vi "WSVCAP SHL FPGA LL I2C Write CLK or DATA Lines.vi"(0 "Bit In":bool, 11 "error in (no error)":errorcluster, 12 "UUT Set (0/1)":u8, 13 "Line":T1, 14 "Socket Mask":u64 format="%08x") -> (15 "error out":errorcluster)   [LabVIEW 2012]
uses:
  Type Defs/WSVCAP SHL I2C Write Line Enum.ctl
  WSVCAP SHL FPGA LL I2C Debug Global.vi
  <vilib>/eio/EIONode/EIONode.xnode
  <vilib>/rvi/eio/common/nirviEmuTemplateMethod_errors.vi
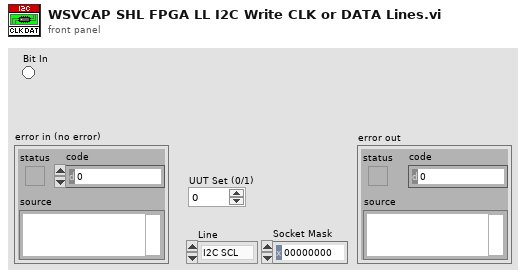
[diagram p1: front panel]
types:
  T1 = typedef "WSVCAP SHL I2C Write Line Enum.ctl" = enum16{"I2C SCL", "I2C SDA"}
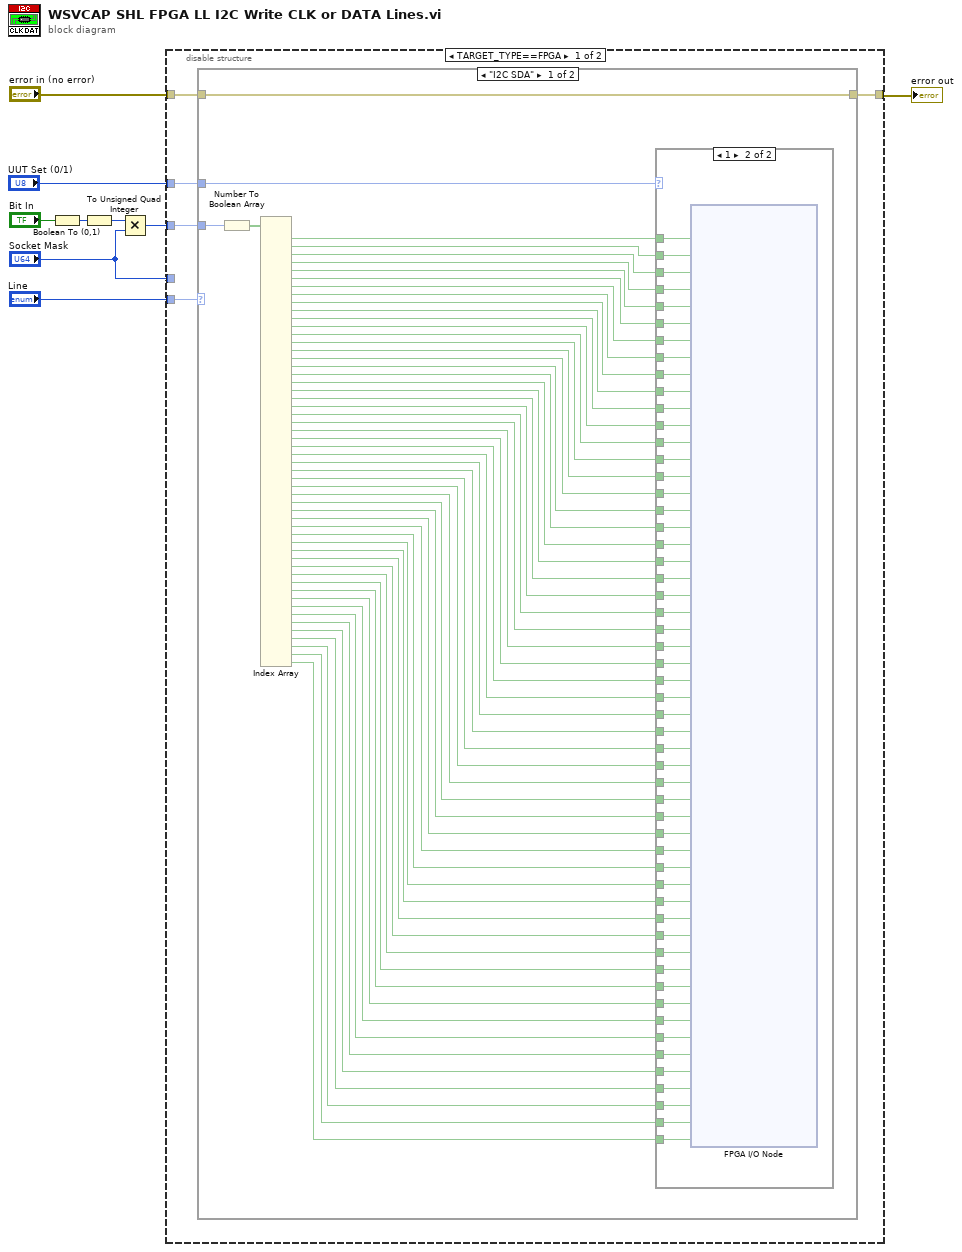
[diagram p0: block diagram]
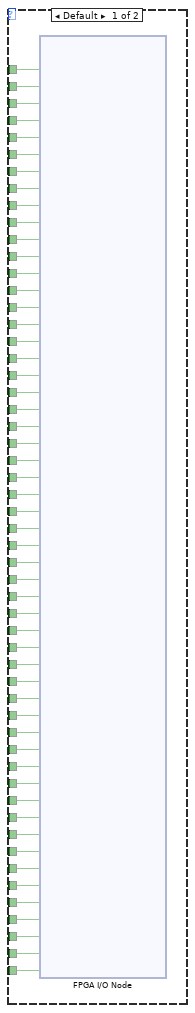
[diagram p2: hidden frame]
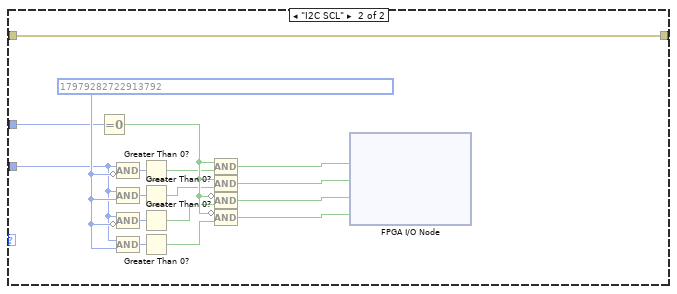
[diagram p3: hidden frame]
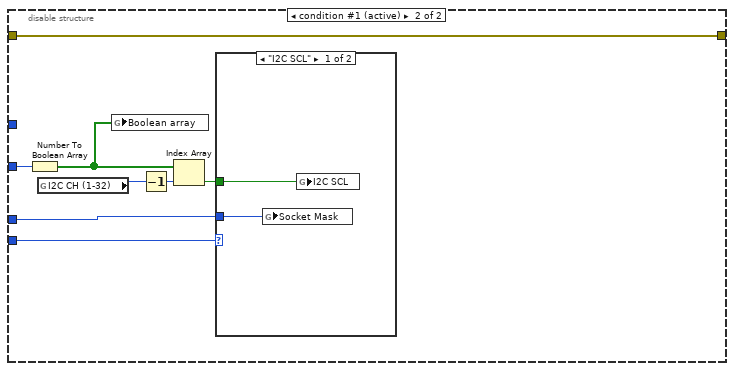
[diagram p4: hidden frame]
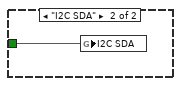
[diagram p5: hidden frame]
diagram:
  n1 = Boolean To (0,1)(Boolean="Bit In") -> (0, 1=w6:i16)
  n2 = To Unsigned Quad Integer(1:w6) -> (0:w5:u64)
  n3 = Multiply(x=w5, y="Socket Mask") -> (x*y=w3:u64)
  n4 = disable-structure shown="TARGET_TYPE==FPGA" {
    disable-tunnel: w3 -> [w14 w200]
    disable-tunnel: "Line" -> [w13 w205]
    disable-tunnel: [w12 w204] -> w8
    disable-tunnel: "error in (no error)" -> [w11 w204]
    disable-tunnel: "Socket Mask" -> [_ w198]
    disable-tunnel: "UUT Set (0/1)" -> [w10 _]
    frame condition #0 {
      n5 = case shown="\"I2C SDA\"" w13 {
        tunnel: w14 -> [w71 w185]
        tunnel: [w70 w197] -> w12
        tunnel: w11 -> [w70 w197]
        tunnel: w10 -> [w33 w186]
        frame "I2C SDA" {
          n6 = Number To Boolean Array(number=w71) -> (Boolean array=w72:bool[])
          n7 = Index Array(array=w72) -> (element #1=w69:bool, element #2=w68:bool, element #3=w67:bool, element #4=w66:bool, element #5=w65:bool, element #6=w64:bool, element #7=w63:bool, element #8=w62:bool, element #9=w61:bool, element #10=w60:bool, element #11=w59:bool, element #12=w58:bool, element #13=w57:bool, element #14=w56:bool, element #15=w55:bool, element #16=w54:bool, element #17=w53:bool, element #18=w52:bool, element #19=w51:bool, element #20=w50:bool, element #21=w49:bool, element #22=w48:bool, element #23=w47:bool, element #24=w46:bool, element #25=w45:bool, element #26=w44:bool, element #27=w43:bool, element #28=w42:bool, element #29=w41:bool, element #30=w40:bool, element #31=w39:bool, element #32=w38:bool, element #33=w37:bool, element #34=w36:bool, element #35=w35:bool, element #36=w34:bool, element #37=w32:bool, element #38=w31:bool, element #39=w30:bool, element #40=w29:bool, element #41=w28:bool, element #42=w27:bool, element #43=w26:bool, element #44=w25:bool, element #45=w24:bool, element #46=w23:bool, element #47=w22:bool, element #48=w21:bool, element #49=w20:bool, element #50=w19:bool, element #51=w18:bool, element #52=w17:bool, element #53=w16:bool, element #54=w15:bool)  [unwired: 54 in]
          n8 = case shown="1" w33 {
            tunnel: w69 -> [w126 w180]
            tunnel: w68 -> [w125 w179]
            tunnel: w67 -> [w124 w178]
            tunnel: w66 -> [w123 w177]
            tunnel: w65 -> [w122 w176]
            tunnel: w64 -> [w121 w175]
            tunnel: w63 -> [w120 w174]
            tunnel: w62 -> [w119 w173]
            tunnel: w61 -> [w118 w172]
            tunnel: w60 -> [w117 w171]
            tunnel: w59 -> [w116 w170]
            tunnel: w58 -> [w115 w169]
            tunnel: w57 -> [w114 w168]
            tunnel: w56 -> [w113 w167]
            tunnel: w55 -> [w112 w166]
            tunnel: w54 -> [w111 w165]
            tunnel: w53 -> [w110 w164]
            tunnel: w52 -> [w109 w163]
            tunnel: w51 -> [w108 w162]
            tunnel: w50 -> [w107 w161]
            tunnel: w49 -> [w106 w160]
            tunnel: w48 -> [w105 w159]
            tunnel: w47 -> [w104 w158]
            tunnel: w46 -> [w103 w157]
            tunnel: w45 -> [w102 w156]
            tunnel: w44 -> [w101 w155]
            tunnel: w43 -> [w100 w154]
            tunnel: w42 -> [w99 w153]
            tunnel: w41 -> [w98 w152]
            tunnel: w40 -> [w97 w151]
            tunnel: w39 -> [w96 w150]
            tunnel: w38 -> [w95 w149]
            tunnel: w37 -> [w94 w148]
            tunnel: w36 -> [w93 w147]
            tunnel: w35 -> [w92 w146]
            tunnel: w34 -> [w91 w145]
            tunnel: w32 -> [w90 w144]
            tunnel: w31 -> [w89 w143]
            tunnel: w30 -> [w88 w142]
            tunnel: w29 -> [w87 w141]
            tunnel: w28 -> [w86 w140]
            tunnel: w27 -> [w85 w139]
            tunnel: w26 -> [w84 w138]
            tunnel: w25 -> [w83 w137]
            tunnel: w24 -> [w82 w136]
            tunnel: w23 -> [w81 w135]
            tunnel: w22 -> [w80 w134]
            tunnel: w21 -> [w79 w133]
            tunnel: w20 -> [w78 w132]
            tunnel: w19 -> [w77 w131]
            tunnel: w18 -> [w76 w130]
            tunnel: w17 -> [w75 w129]
            tunnel: w16 -> [w74 w128]
            tunnel: w15 -> [w73 w127]
            frame Default {
              n9 = xnode "FPGA I/O Node"("I2C_SDA_C1_S1"=w126, "I2C_SDA_C1_S2"=w125, "I2C_SDA_C1_S3"=w124, "I2C_SDA_C1_S4"=w123, "I2C_SDA_C1_S5"=w122, "I2C_SDA_C1_S6"=w121, "I2C_SDA_C1_S7"=w120, "I2C_SDA_C1_S8"=w119, "I2C_SDA_C1_S9"=w118, "I2C_SDA_C1_S10"=w117, "I2C_SDA_C1_S11"=w116, "I2C_SDA_C1_S12"=w115, "I2C_SDA_C1_S13"=w114, "I2C_SDA_C1_S14"=w113, "I2C_SDA_C1_S15"=w112, "I2C_SDA_C1_S16"=w111, "I2C_SDA_C1_S17"=w110, "I2C_SDA_C1_S18"=w109, "I2C_SDA_C2_S1"=w108, "I2C_SDA_C2_S2"=w107, "I2C_SDA_C2_S3"=w106, "I2C_SDA_C2_S4"=w105, "I2C_SDA_C2_S5"=w104, "I2C_SDA_C2_S6"=w103, "I2C_SDA_C2_S7"=w102, "I2C_SDA_C2_S8"=w101, "I2C_SDA_C2_S9"=w100, "I2C_SDA_C2_S10"=w99, "I2C_SDA_C2_S11"=w98, "I2C_SDA_C2_S12"=w97, "I2C_SDA_C2_S13"=w96, "I2C_SDA_C2_S14"=w95, "I2C_SDA_C2_S15"=w94, "I2C_SDA_C2_S16"=w93, "I2C_SDA_C2_S17"=w92, "I2C_SDA_C2_S18"=w91, "I2C_SDA_C3_S1"=w90, "I2C_SDA_C3_S2"=w89, "I2C_SDA_C3_S3"=w88, "I2C_SDA_C3_S4"=w87, "I2C_SDA_C3_S5"=w86, "I2C_SDA_C3_S6"=w85, "I2C_SDA_C3_S7"=w84, "I2C_SDA_C3_S8"=w83, "I2C_SDA_C3_S9"=w82, "I2C_SDA_C3_S10"=w81, "I2C_SDA_C3_S11"=w80, "I2C_SDA_C3_S12"=w79, "I2C_SDA_C3_S13"=w78, "I2C_SDA_C3_S14"=w77, "I2C_SDA_C3_S15"=w76, "I2C_SDA_C3_S16"=w75, "I2C_SDA_C3_S17"=w74, "I2C_SDA_C3_S18"=w73) -> ()  [unwired: 55 in, 55 out]
            }
            frame 1 {
              n10 = xnode "FPGA I/O Node"("I2C_SDA_C1_S19"=w180, "I2C_SDA_C1_S20"=w179, "I2C_SDA_C1_S21"=w178, "I2C_SDA_C1_S22"=w177, "I2C_SDA_C1_S23"=w176, "I2C_SDA_C1_S24"=w175, "I2C_SDA_C1_S25"=w174, "I2C_SDA_C1_S26"=w173, "I2C_SDA_C1_S27"=w172, "I2C_SDA_C1_S28"=w171, "I2C_SDA_C1_S29"=w170, "I2C_SDA_C1_S30"=w169, "I2C_SDA_C1_S31"=w168, "I2C_SDA_C1_S32"=w167, "I2C_SDA_C1_S33"=w166, "I2C_SDA_C1_S34"=w165, "I2C_SDA_C1_S35"=w164, "I2C_SDA_C1_S36"=w163, "I2C_SDA_C2_S19"=w162, "I2C_SDA_C2_S20"=w161, "I2C_SDA_C2_S21"=w160, "I2C_SDA_C2_S22"=w159, "I2C_SDA_C2_S23"=w158, "I2C_SDA_C2_S24"=w157, "I2C_SDA_C2_S25"=w156, "I2C_SDA_C2_S26"=w155, "I2C_SDA_C2_S27"=w154, "I2C_SDA_C2_S28"=w153, "I2C_SDA_C2_S29"=w152, "I2C_SDA_C2_S30"=w151, "I2C_SDA_C2_S31"=w150, "I2C_SDA_C2_S32"=w149, "I2C_SDA_C2_S33"=w148, "I2C_SDA_C2_S34"=w147, "I2C_SDA_C2_S35"=w146, "I2C_SDA_C2_S36"=w145, "I2C_SDA_C3_S19"=w144, "I2C_SDA_C3_S20"=w143, "I2C_SDA_C3_S21"=w142, "I2C_SDA_C3_S22"=w141, "I2C_SDA_C3_S23"=w140, "I2C_SDA_C3_S24"=w139, "I2C_SDA_C3-S25"=w138, "I2C_SDA_C3_S26"=w137, "I2C_SDA_C3_S27"=w136, "I2C_SDA_C3_S28"=w135, "I2C_SDA_C3_S29"=w134, "I2C_SDA_C3_S30"=w133, "I2C_SDA_C3_S31"=w132, "I2C_SDA_C3_S32"=w131, "I2C_SDA_C3_S33"=w130, "I2C_SDA_C3_S34"=w129, "I2C_SDA_C3_S35"=w128, "I2C_SDA_C3_S36"=w127) -> ()  [unwired: 55 in, 55 out]
            }
          }
        }
        frame "I2C SCL" {
          w187 = u64 17979282722913792
          n11 = Equal To 0?(x=w186) -> (x = 0?=w196:bool)
          n12 = Compound Arithmetic op=AND(w185, invert w187) -> (w195:u64)
          n13 = Compound Arithmetic op=AND(w185, w187) -> (w193:u64)
          n14 = Compound Arithmetic op=AND(w185, invert w187) -> (w192:u64)
          n15 = Compound Arithmetic op=AND(w185, w187) -> (w191:u64)
          n16 = Greater Than 0?(x=w195) -> (x > 0?=w194:bool)
          n17 = Greater Than 0?(x=w193) -> (x > 0?=w190:bool)
          n18 = Greater Than 0?(x=w192) -> (x > 0?=w189:bool)
          n19 = Greater Than 0?(x=w191) -> (x > 0?=w188:bool)
          n20 = Compound Arithmetic op=AND(w196, w194) -> (w184:bool)
          n21 = Compound Arithmetic op=AND(w196, w190) -> (w183:bool)
          n22 = Compound Arithmetic op=AND(invert w196, w189) -> (w182:bool)
          n23 = Compound Arithmetic op=AND(invert w196, w188) -> (w181:bool)
          n24 = xnode "FPGA I/O Node"("I2C_SCL_S1-9"=w184, "I2C_SCL_S10-18"=w183, "I2C_SCL_S19-27"=w182, "I2C_SCL_S28-36"=w181) -> ()  [unwired: 5 in, 5 out]
        }
      }
    }
    frame condition #1 (active) {
      n25 = Number To Boolean Array(number=w200) -> (Boolean array=w199:bool[])
      n26 = global read "WSVCAP SHL FPGA LL I2C Debug Global.vi" "I2C CH (1-32)"() -> (w202:i32)
      n27 = global write "WSVCAP SHL FPGA LL I2C Debug Global.vi" "Boolean array"(w199) -> ()
      n28 = Decrement(x=w202) -> (x-1=w201:i32)
      n29 = Index Array(array=w199, index=w201) -> (element=w203:bool)
      n30 = case shown="\"I2C SCL\"" w205 {
        tunnel: w203 -> [w207 w208]
        tunnel: w198 -> [w206 _]
        frame "I2C SCL" {
          n31 = global write "WSVCAP SHL FPGA LL I2C Debug Global.vi" "Socket Mask"(w206) -> ()
          n32 = global write "WSVCAP SHL FPGA LL I2C Debug Global.vi" "I2C SCL"(w207) -> ()
        }
        frame "I2C SDA" {
          n33 = global write "WSVCAP SHL FPGA LL I2C Debug Global.vi" "I2C SDA"(w208) -> ()
        }
      }
    }
  }
  "error out" <- w8
